vi "Test_InitProgress.vi"() -> ()   [LabVIEW 2011]
panel:
  in  "InitProgRef":refnum<vi>
  in  "%Ref":refnum<vi>
  in  "EscapeRef":refnum<vi>
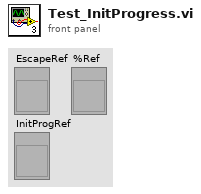
[diagram p1: front panel]
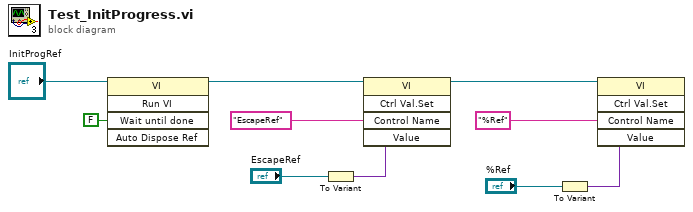
[diagram p0: block diagram]
diagram:
  n1 = invoke class="VI" method="Run VI"(reference="InitProgRef", "Wait until done"=FALSE ("Wait Until Done")) -> (reference out=w4:refnum<vi>)  [unwired: 3 in, 4 out]
  n2 = To Variant(anything="EscapeRef") -> (Variant=w8:variant)
  n3 = invoke class="VI" method="Ctrl Val.Set"(reference=w4, "Control Name"="EscapeRef" ("Name"), "Value"=w8) -> (reference out=w7:refnum<vi>)  [unwired: 2 in, 4 out]
  n4 = To Variant(anything="%Ref") -> (Variant=w6:variant)
  n5 = invoke class="VI" method="Ctrl Val.Set"(reference=w7, "Control Name"="%Ref" ("Name"), "Value"=w6) -> ()  [unwired: 2 in, 5 out]
